vi "DBserverConnect.vi"() -> (0 "Connection Out":refnum<k7>)   [LabVIEW 2025]
uses:
  <vilib>/Utility/config.llb/NI_LVConfig.lvlib
  <vilib>/Utility/config.llb/Read Key (String).vi
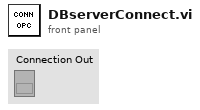
[diagram p1: front panel]
types:
  T1 = typedef "NI_LVConfig.lvlib/Config Data RefNum.ctl" = refnum<k1>
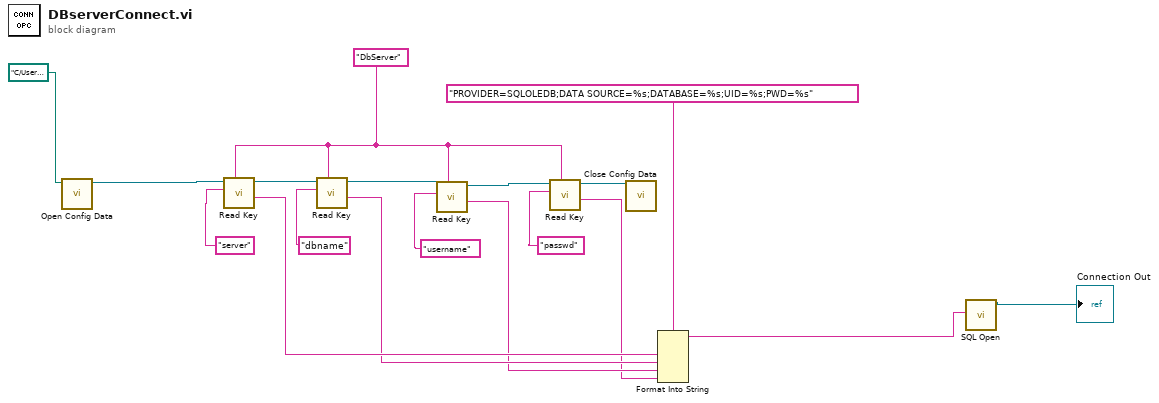
[diagram p0: block diagram]
diagram:
  w13 = "DbServer"
  n1 = call <vilib>:"Open Config Data.vi"("configuration file path"=path "C:/Users/magne/OneDrive/Dokumenter/Skole/IIA2017-1 26V Industrial Information Technology/Assignments/SCADA Assignment/02 Files/Task 3/settings.ini") -> ("refnum"=w17:T1)  [unwired: 8 in, 2 out]
  n2 = call-poly <vilib>:"Read Key.vi"("section"=w13, "key"="server", "refnum"=w17) -> ("value"=w6:string, "refnum out"=w16:T1)  [unwired: 5 in, 2 out]
  n3 = call-poly <vilib>:"Read Key.vi"("section"=w13, "key"="dbname", "refnum"=w16) -> ("value"=w5:string, "refnum out"=w15:T1)  [unwired: 5 in, 2 out]
  n4 = call-poly <vilib>:"Read Key.vi"("section"=w13, "key"="username", "refnum"=w15) -> ("value"=w4:string, "refnum out"=w14:T1)  [unwired: 5 in, 2 out]
  n5 = call-poly <vilib>:"Read Key.vi"("section"=w13, "key"="passwd", "refnum"=w14) -> ("value"=w3:string, "refnum out"=w8:T1)  [unwired: 5 in, 2 out]
  n6 = call <vilib>:"Close Config Data.vi"("refnum"=w8) -> ()  [unwired: 9 in, 2 out]
  n7 = Format Into String(format string="PROVIDER=SQLOLEDB;DATA SOURCE=%s;DATABASE=%s;UID=%s;PWD=%s", w6, w5, w4, w3) -> (resulting string=w2:string)  [unwired: 2 in, 1 out]
  n8 = call <vilib>:"SQL Open.vi"("ConnectionString In"=w2) -> ("Connection Out"=→"Connection Out":refnum<k7>)  [unwired: 17 in, 1 out]
